vi "Execute.vi"(8 "error in (no error)":errorcluster, 11 "Node in":refnum<class "bt_Parallel_Interleaved.lvclass">) -> (0 "error out":errorcluster, 1 "Status":T1, 3 "Node out":refnum<class "bt_Parallel_Interleaved.lvclass">)   [LabVIEW 2021, in "BT.lvlib" / "bt_Parallel_Interleaved.lvclass"]
uses:
  bt_Parallel_Interleaved.lvclass
  C:/Users/Tim/Documents/GitHub/LV_Behaviour_Tree/Source/Support/Nodes/Composites/abs_Parallel/bt_Parallel.lvclass
  C:/Users/Tim/Documents/GitHub/LV_Behaviour_Tree/Source/Support/Nodes/Composites/abs_Composite/bt_Composite.lvclass
  abs_Node/Status.ctl
  abs_Composite/bt_Composite.lvclass/bt_Composite.ctl
  abs_Composite/Properties/Read Index.vi
  abs_Composite/Properties/Read Num Nodes.vi
  abs_Composite/Properties/Write Index.vi
  abs_Parallel/bt_Parallel.lvclass
  bt_Parallel_Interleaved.lvclass/bt_Parallel_Interleaved.ctl
  abs_Node/bt_Node.lvclass
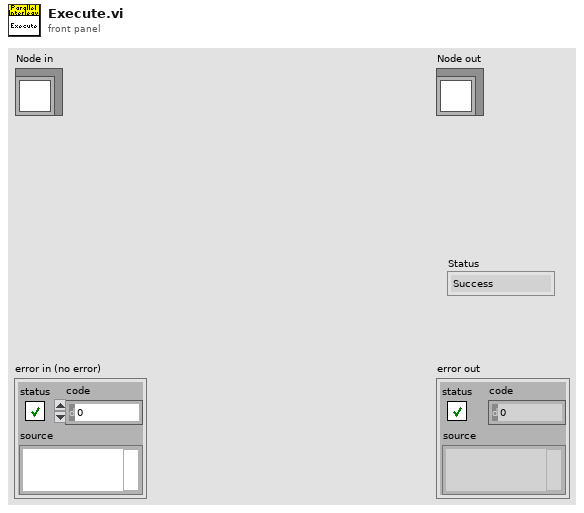
[diagram p1: front panel]
types:
  T1 = typedef "BT.lvlib/bt_Node.lvclass/Status.ctl" = enum16{"Success", "Failure", "Running"}
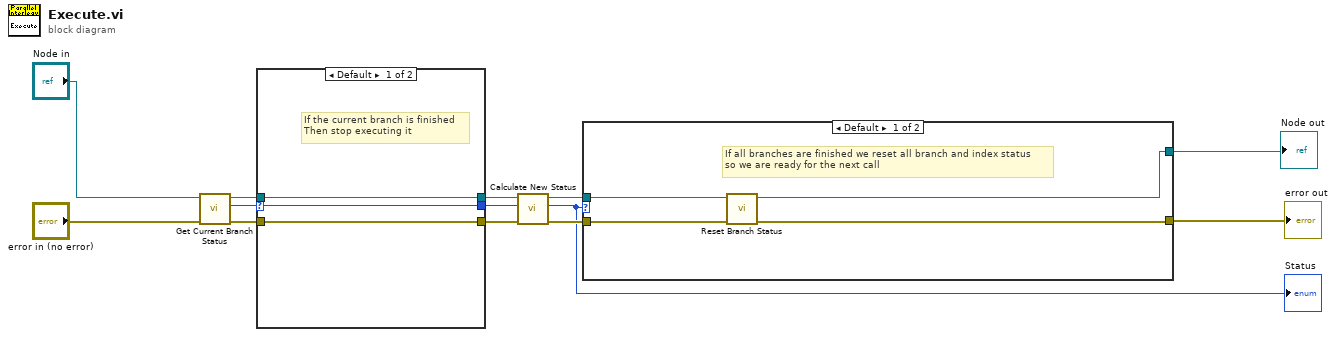
[diagram p0: block diagram]
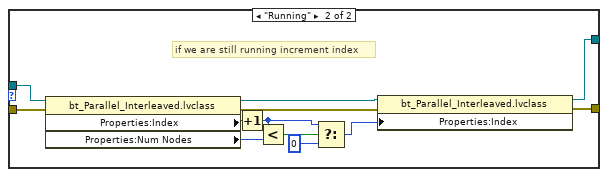
[diagram p2: hidden frame]
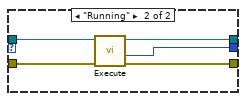
[diagram p3: hidden frame]
diagram:
  n1 = call "Get Current Branch Status.vi"("error in (no error)"="error in (no error)", "abs_Parallel in"="Node in") -> ("error out"=w9:errorcluster, "Previous Status"=w7:T1, "abs_Parallel out"=w8:refnum<class "bt_Parallel_Interleaved.lvclass">)  [unwired: 7 in]
  n2 = case shown="Default" w7 {
    selector: w7 -> [w14 _]
    tunnel: [w16 w19] -> w4
    tunnel: [w15 w18] -> w6
    tunnel: w8 -> [w16 w21]
    tunnel: w9 -> [w15 w20]
    tunnel: [w14 w17] -> w1
    frame Default {
      # "If the current branch is finished\nThen stop executing it"
    }
    frame "Running" {
      n3 = call-parent "Execute.vi"("error in (no error)"=w20, "Node in"=w21) -> ("error out"=w18:errorcluster, "Status"=w17:T1, "Node out"=w19:refnum<class "bt_Parallel_Interleaved.lvclass">)  [unwired: 7 in]
    }
  }
  n4 = call "Calculate New Status.vi"("error in (no error)"=w6, "New Status"=w1, "abs_Parallel in"=w4) -> ("error out"=w5:errorcluster, "Overall Status"=w2:T1, "abs_Parallel out"=w3:refnum<class "bt_Parallel_Interleaved.lvclass">)  [unwired: 6 in]
  "Status" <- w2
  n5 = case shown="Default" w2 {
    tunnel: [w22 w37] -> w11
    tunnel: [w23 w36] -> w10
    tunnel: w3 -> [w25 w35]
    tunnel: w5 -> [w24 w32]
    frame Default {
      # "If all branches are finished we reset all branch and index status\nso we are ready for the next call"
      n6 = call "Reset Branch Status.vi"("error in (no error)"=w24, "bt_Parallel in"=w25) -> ("error out"=w22:errorcluster, "bt_Parallel out"=w23:refnum<class "bt_Parallel_Interleaved.lvclass">)  [unwired: 8 in]
    }
    frame "Running" {
      # "if we are still running increment index"
      n7 = property class="bt_Parallel_Interleaved.lvclass"(reference=w35, error in=w32) -> (reference out=w34:refnum<class "bt_Parallel_Interleaved.lvclass">, error out=w31:errorcluster, "Properties:Index"=w30:i32, "Properties:Num Nodes"=w29:i32)
      n8 = Increment(x=w30) -> (x+1=w27:i32)
      n9 = Less?(x=w27, y=w29) -> (x < y?=w28:bool)
      n10 = Select(t=w27, s=w28, f=0) -> (s? t:f=w33:i32)
      n11 = property class="bt_Parallel_Interleaved.lvclass"(reference=w34, error in=w31, "Properties:Index"=w33) -> (reference out=w36:refnum<class "bt_Parallel_Interleaved.lvclass">, error out=w37:errorcluster)
    }
  }
  "error out" <- w11
  "Node out" <- w10
